vi "AddQ_Provider_OnPopupMenu.vi"(11 "objects":T1[](array[typedef])) -> ()   [LabVIEW 2017, in "G#IDE.lvlib"]
uses:
  <resource>/Framework/Providers/AddQ/G#IDE/G#IDE.lvlib
  <resource>/Framework/Providers/API/ItemRef.ctl
  <resource>/Framework/Providers/API/mxLvMenuItem.ctl
  <resource>/Framework/Providers/AddQ/G#IDE/support/ProviderLib/ProviderLib.lvlib
panel:
  out "error out":errorcluster
  in  "error in":errorcluster
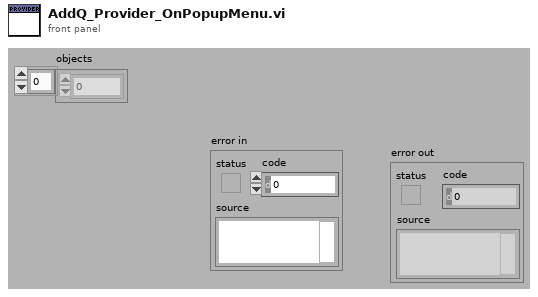
[diagram p1: front panel]
types:
  T1 = typedef "ItemRef.ctl" = u64
  T2 = typedef "mxLvMenuItem.ctl" = cluster{"Menu Name":string, "Description":string, "Icon File Name":path, "Menu Tag":string, "Enabled":bool, "Checked":bool, "Separator":bool, "Batchable":bool, "Weight":i32, "Batch Mode (Ignored if Not Batchable)":enum32{"Show If All Items Support Command", "Show If Any Items Support Command"}, "Menu Location":enum32{"<None>", "Project", "Project / Build Specifications", "Tools", "Tools / Source Control", "Tools / Real-Time Module", "Help"}, "Exclude From Getting Started Window Menu":bool}
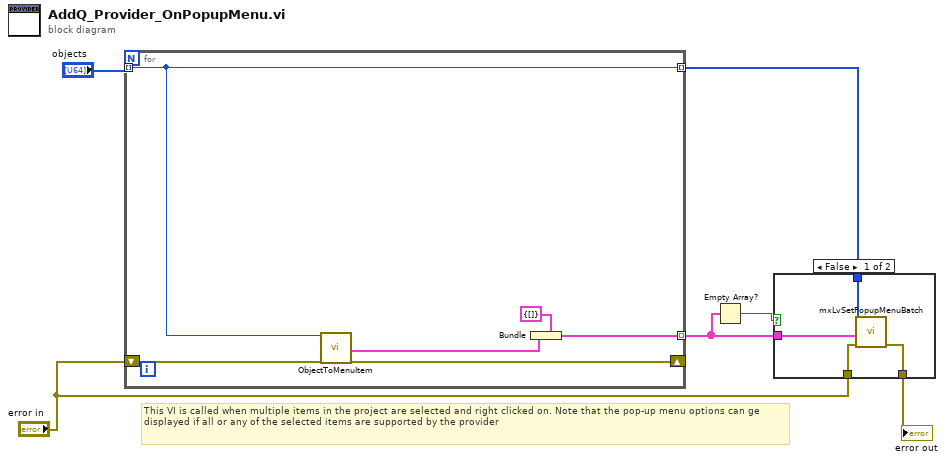
[diagram p0: block diagram]
diagram:
  # "This VI is called when multiple items in the project are selected and right clicked on. Note that the pop-up menu options can ge displayed if all or any of the selected items are supported by the provider"
  n1 = for {
    tunnel: "objects" -> [w8] mode=indexing
    tunnel: [w8] -> w4 mode=indexing
    tunnel: [w11] -> w2 mode=indexing
    shift-right: [w9] -> _
    shift-left: "error in" -> [w10]
    n2 = call <resource>:"ObjectToMenuItem.vi"("Object"=w8, "error in (no error)"=w10) -> ("Popup Menu Items"=w7:T2[], "error out"=w9:errorcluster)  [unwired: 15 in, 1 out]
    n3 = Bundle(cluster=cluster{"Popup Menu Items":T2[]} {"Popup Menu Items"=[]} ("y"), "Popup Menu Items"=w7) -> (w11:cluster{"Popup Menu Items":T2[]})
  }
  n4 = Empty Array?(array=w2) -> (empty?=w1:bool)
  n5 = case shown="False" w1 {
    tunnel: [w16 w17] -> w6
    tunnel: w4 -> [w15 _]
    tunnel: w2 -> [w14 _]
    tunnel: "error in" -> [w13 w17]
    frame False {
      n6 = call <resource>:"mxLvSetPopupMenuBatch.vi"("error in"=w13, "Menu Items"=w14, "Items"=w15) -> ("error out"=w16:errorcluster)  [unwired: 7 in, 1 out]
    }
    frame True {
    }
  }
  "error out" <- w6
